vi "Create Mecanum Wheel.vi"(6 "motor communication":refnum<class "NI_Robotics_Motor Communication.lvclass">, 7 "roller orientation":T1 items=["Left", "Right"], 8 "error in (no error)":errorcluster, 10 "wheel name":string, 11 "wheel parameters":T2={"wheel radius"=1.0, "gear ratio"=1.0, "forward rotation direction"=0} {"forward rotation direction" items=["Clockwise", "Counterclockwise"]}) -> (0 "error out":errorcluster, 3 "mecanum wheel out":refnum<class "NI_Robotics_Mecanum Wheel.lvclass">)   [LabVIEW 2017, in "NI_Robotics_Mecanum Wheel.lvclass"]
doc: "Creates a wheel of the type you specify that you can add to a steering frame. You must manually select the polymorphic instance to use."
uses:
  <vilib>/robotics/Steering/Mecanum Wheel/NI_Robotics_Mecanum Wheel.lvclass
  c:/Program Files (x86)/National Instruments/LabVIEW 2017/vi.lib/robotics/Steering/Wheel/NI_Robotics_Wheel.lvclass
  <vilib>/robotics/Steering/Wheel/Wheel Parameters.ctl
  <vilib>/robotics/Steering/Wheel/Rotation Direction.ctl
  <vilib>/robotics/Actuation/Motor Communication/NI_Robotics_Motor Communication.lvclass
  <vilib>/robotics/Steering/Mecanum Wheel/Roller Orientation.ctl
  <vilib>/robotics/Actuation/Motor Communication/NI_Robotics_Motor Communication.lvclass/NI_Robotics_Motor Communication.ctl
  <vilib>/robotics/Steering/Wheel/NI_Robotics_Wheel.lvclass/NI_Robotics_Wheel.ctl
  <vilib>/robotics/Steering/Mecanum Wheel/NI_Robotics_Mecanum Wheel.lvclass/NI_Robotics_Mecanum Wheel.ctl
  <vilib>/robotics/Actuation/Motor Communication/Get Initialized State.vi
  <vilib>/robotics/Actuation/Motor Communication Val/NI_Robotics_Motor Communication Val.lvclass
  c:/Program Files (x86)/National Instruments/LabVIEW 2017/vi.lib/robotics/Actuation/Motor Communication/NI_Robotics_Motor Communication.lvclass
  <vilib>/robotics/Actuation/Motor Communication Val/Initialize Motor Communication Val.vi
  <vilib>/robotics/Steering/Wheel/NI_Robotics_Wheel.lvclass
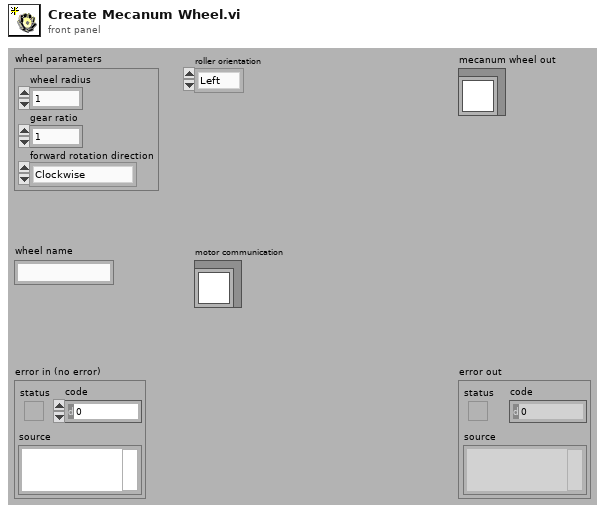
[diagram p1: front panel]
types:
  T1 = typedef "NI_Robotics_Mecanum Wheel.lvclass/Roller Orientation.ctl" = u16
  T2 = typedef "NI_Robotics_Wheel.lvclass/Wheel Parameters.ctl" = cluster{"wheel radius":dbl, "gear ratio":dbl, "forward rotation direction":T3}
  T3 = typedef "NI_Robotics_Wheel.lvclass/Rotation Direction.ctl" = u16
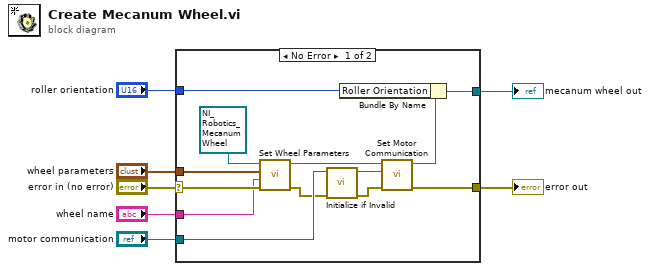
[diagram p0: block diagram]
diagram:
  n1 = case shown="No Error" "error in (no error)" {
    selector: "error in (no error)" -> [w18 w21]
    tunnel: [w12 w21] -> w6
    tunnel: "wheel parameters" -> [w19 _]
    tunnel: "roller orientation" -> [w17 _]
    tunnel: "motor communication" -> [w11 _]
    tunnel: [w16 _] -> w2
    tunnel: "wheel name" -> [w15 _]
    frame No Error {
      n2 = call <vilib>:"Set Wheel Parameters.vi"("error in (no error)"=w18, "wheel name"=w15, "wheel parameters"=w19, "wheel in"=refnum<class "NI_Robotics_Mecanum Wheel.lvclass"> refnum ("Mecanum Wheel in")) -> ("error out"=w9:errorcluster, "wheel out"=w14:refnum<class "NI_Robotics_Mecanum Wheel.lvclass">)  [unwired: 6 in]
      n3 = call <vilib>:"Initialize if Invalid.vi"("error in (no error)"=w9, "motor communication in"=w11) -> ("error out"=w8:errorcluster, "motor communication out"=w10:refnum<class "NI_Robotics_Motor Communication.lvclass">)  [unwired: 7 in, 1 out]
      n4 = call <vilib>:"Set Motor Communication.vi"("error in (no error)"=w8, "motor communication"=w10, "wheel in"=w14) -> ("error out"=w12:errorcluster, "wheel out"=w13:refnum<class "NI_Robotics_Mecanum Wheel.lvclass">)  [unwired: 7 in]
      n5 = Bundle By Name(cluster=w13, "Roller Orientation"=w17) -> (w16:refnum<class "NI_Robotics_Mecanum Wheel.lvclass">)
    }
    frame Error {
    }
  }
  "error out" <- w6
  "mecanum wheel out" <- w2
